vi "Main Host MSS test.vi"() -> ()   [LabVIEW 2023]
uses:
  MSS/MSS Host Actor/MSS Host Actor.lvclass
  C:/Program Files/National Instruments/LabVIEW 2023/vi.lib/ActorFramework/Actor/Actor.lvclass
  <vilib>/ni/Actors/Network Endpoint Actors/Protocols/Network Stream Strategy/Network Stream/Network Stream.lvclass/Network Stream.ctl
  <vilib>/ni/Actors/Network Endpoint Actors/Protocols/Network Stream Strategy/Network Stream Initiator/Network Stream Initiator.lvclass/Network Stream Initiator.ctl
  MSS/MSS Host Actor/MSS Host Actor.lvclass/MSS Host Actor.ctl
  <vilib>/ni/Actors/Network Endpoint Actors/Protocols/Network Stream Strategy/Network Stream/Write Buffer Size.vi
  <vilib>/ni/Actors/Network Endpoint Actors/Protocols/Network Stream Strategy/Network Stream/Write Name.vi
  <vilib>/ni/Actors/Network Endpoint Actors/Protocols/Network Stream Strategy/Network Stream Initiator/Network Stream Initiator.lvclass
  C:/Program Files/National Instruments/LabVIEW 2023/vi.lib/ni/Actors/Network Endpoint Actors/Protocols/Network Stream Strategy/Network Stream/Network Stream.lvclass
  C:/Program Files/National Instruments/LabVIEW 2023/vi.lib/ni/Actors/Network Endpoint Actors/Abstract Classes/Message Stream/Message Stream.lvclass
  <vilib>/ActorFramework/Actor/Actor.lvclass
panel:
  out "error out":errorcluster
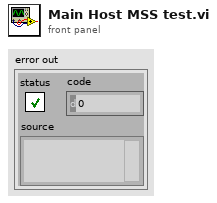
[diagram p1: front panel]
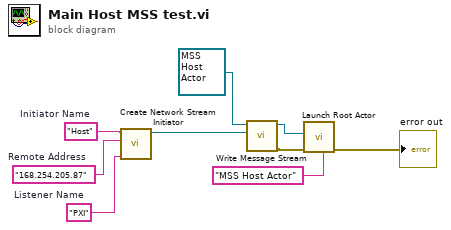
[diagram p0: block diagram]
diagram:
  w7 = "PXI"  # Listener Name
  w8 = "168.254.205.87"  # Remote Address
  w9 = "Host"  # Initiator Name
  n1 = call <vilib>:"Create Network Stream Initiator.vi"("Remote Context"=w7, "Remote Address"=w8, "Name"=w9) -> ("Network Stream Initiator out"=w5:refnum<class "Network Stream Initiator.lvclass">)  [unwired: 8 in]
  n2 = call "Write Message Stream.vi"("Message Stream.lvclass"=w5, "MSS Host Actor in"=refnum<class "MSS Host Actor.lvclass"> refnum ("MSS Host Actor.lvlib:MSS Host Actor.lvclass")) -> ("error out"=w4:errorcluster, "MSS Host Actor out"=w2:refnum<class "MSS Host Actor.lvclass">)  [unwired: 8 in]
  n3 = call <vilib>:"Launch Root Actor.vi"("Debug Alias"="MSS Host Actor", "error in (no error)"=w4, "Actor"=w2) -> ("error out"=→"error out":errorcluster)  [unwired: 7 in, 1 out]
